vi "Resume_Sequence.vi"(2 "Alias Table":string[][](array[string]), 3 "Sequence":cluster{string, string[], dbl[], dbl}[](array[cluster])) -> (0 "Cancelled":bool, 1 "Start Event Value":i32)   [LabVIEW 2011]
doc: "This modal VI functions as a popup, displaying the step at which the previous growth sequence run was paused, and allowing the user to continue on from this step, or at the user's discretion, any other step in the growth sequence."
uses:
  low_level_proc/globals.vi
panel:
  out "Last Event When Paused:":string
  in  "Cancel":bool
  in  "OK":bool
  in  "Start Event":string(combo)
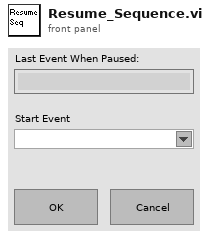
[diagram p1: front panel]
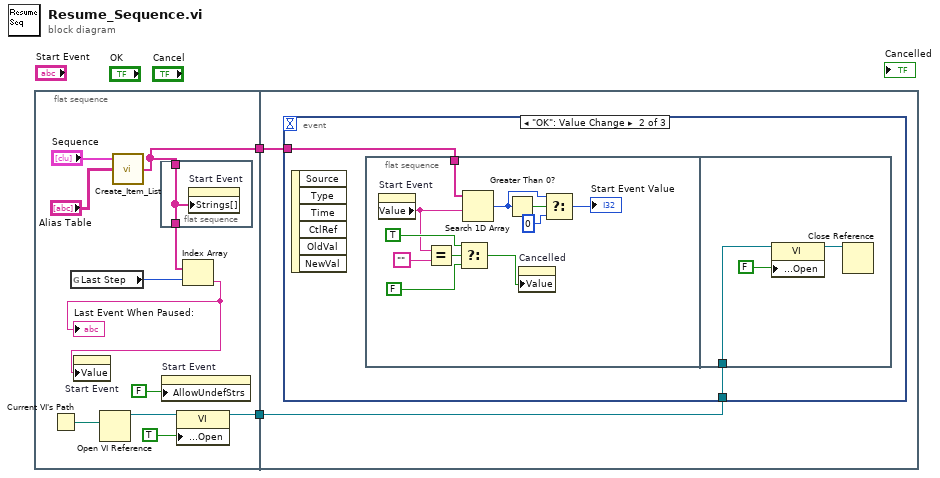
[diagram p0: block diagram]
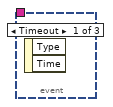
[diagram p2: hidden frame]
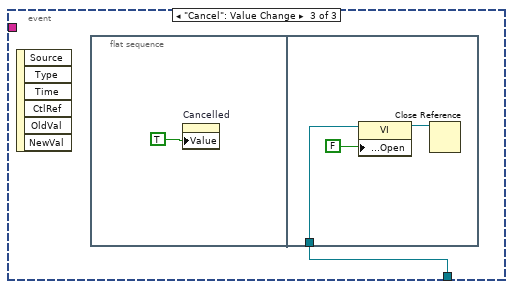
[diagram p3: hidden frame]
diagram:
  n1 = flat-sequence {
    tunnel: [w12] -> w2
    tunnel: [w5] -> w1
    tunnel: w2 -> [w16]
    tunnel: w1 -> [w15]
    frame #0 {
      n2 = Current VI's Path() -> (path=w10:path)
      n3 = global read "globals.vi" "Last Step"() -> (w6:i32)
      n4 = Open VI Reference(vi path=w10) -> (vi reference=w11:refnum<vi>)  [unwired: 1 in, 5 out]
      n5 = call "Create_Item_List.vi"("Alias Table"="Alias Table", "Sequence"="Sequence") -> ("Item List"=w5:string[])  [unwired: 1 in]
      n6 = flat-sequence {
        tunnel: w5 -> [w14]
        tunnel: [w14] -> w4
        frame #0 {
          n7 = property on="Start Event" class="CmbBox"("Strings[]"=w14) -> ()  [unwired: 2 in, 2 out]
        }
      }
      n8 = property on="Start Event" class="CmbBox"("AllowUndefStrs"=FALSE ("Allow Undefined Strings")) -> ()  [unwired: 2 in, 2 out]
      n9 = property class="VI"(reference=w11, "Front Panel.Open"=TRUE ("Front Panel Window:Open")) -> (reference out=w12:refnum<vi>)  [unwired: 1 in, 1 out]
      n10 = Index Array(array=w4, index=w6) -> (element=w3:string)
      "Last Event When Paused:" <- w3
      n11 = property on="Start Event" class="CmbBox"("Value"=w3) -> ()  [unwired: 2 in, 2 out]
    }
    frame #1 {
      n12 = event shown="[1] \"OK\": Value Change" {
        selector: _ -> [_ _ _]
        dyn-events: _ -> [_ _ _]
        timeout: _ -> [_ _ _]
        tunnel: w16 -> [_ w18 w33]
        tunnel: w15 -> [_ w17 _]
        event Timeout {
          n13 = event-data() -> ()  [unwired: 3 out]
        }
        event "OK": Value Change {
          n14 = event-data() -> ()  [unwired: 7 out]
          n15 = flat-sequence {
            tunnel: w17 -> [w24]
            tunnel: w18 -> [w31]
            frame #0 {
              n16 = property on="Start Event" class="CmbBox"() -> ("Value"=w23:string)  [unwired: 2 in, 2 out]
              n17 = Equal?(x=w23, y="") -> (x = y?=w26:bool)
              n18 = Select(t=TRUE ("Cancelled"), s=w26, f=FALSE) -> (s? t:f=w27:bool)
              n19 = Search 1D Array(1D array=w24, element=w23) -> (index of element=w21:i32)  [unwired: 1 out]
              n20 = Greater Than 0?(x=w21) -> (x > 0?=w22:bool)
              n21 = property on="Cancelled" class="Bool (strict)"("Value"=w27) -> ()  [unwired: 2 in, 2 out]
              n22 = Select(t=w21, s=w22, f=0) -> (s? t:f=→"Start Event Value":i32)
            }
            frame #1 {
              n23 = property class="VI"(reference=w31, "Front Panel.Open"=FALSE ("Front Panel Window:Open")) -> (reference out=w30:refnum<vi>)  [unwired: 1 in, 1 out]
              n24 = Close Reference(reference=w30) -> ()  [unwired: 1 in, 1 out]
            }
          }
        }
        event "Cancel": Value Change {
          n25 = event-data() -> ()  [unwired: 7 out]
          n26 = flat-sequence {
            tunnel: w33 -> [w36]
            frame #0 {
              n27 = property on="Cancelled" class="Bool (strict)"("Value"=TRUE ("Cancelled")) -> ()  [unwired: 2 in, 2 out]
            }
            frame #1 {
              n28 = property class="VI"(reference=w36, "Front Panel.Open"=FALSE ("Front Panel Window:Open")) -> (reference out=w35:refnum<vi>)  [unwired: 1 in, 1 out]
              n29 = Close Reference(reference=w35) -> ()  [unwired: 1 in, 1 out]
            }
          }
        }
      }
    }
  }
